vi "step function.vi"() -> ()   [LabVIEW 2023]
panel:
  out "s? t:f":dbl
  in  "x":dbl
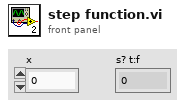
[diagram p1: front panel]
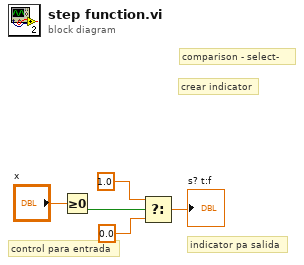
[diagram p0: block diagram]
diagram:
  # "control para entrada"
  # "indicator pa salida"
  # "crear indicator"
  # "comparison - select-"
  n1 = Greater Or Equal To 0?(x="x") -> (x >= 0?=w3:bool)
  n2 = Select(t=1.0, s=w3, f=0.0) -> (s? t:f=→"s? t:f":dbl)
